vi "VGF Data.vi"(10 "Data":T1, 11 "Accion":enum16{"Read", "Set_data"}(ring)) -> (2 "Data 2":T1)   [LabVIEW 2019, in "Analisis.lvlib"]
doc: "FGV dedicated to storage momentarily the data in the analisis interface. This data is obtained in SAVE_DB_SQLite module to storage in the database"
uses:
  Analisis.lvlib
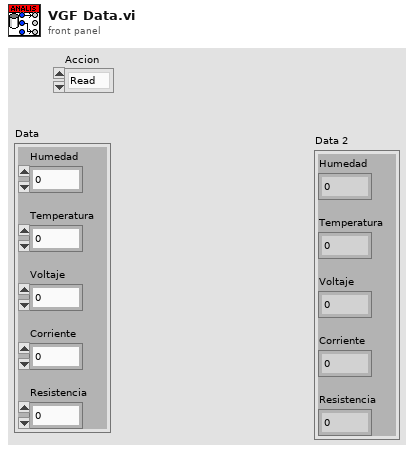
[diagram p1: front panel]
types:
  T1 = cluster{"Humedad":dbl, "Temperatura":dbl, "Voltaje":dbl, "Corriente":dbl, "Resistencia":i32}
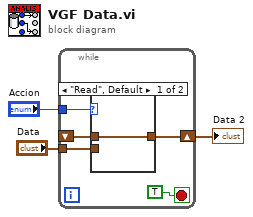
[diagram p0: block diagram]
diagram:
  n1 = while {
    tunnel: "Accion" -> [w8]
    tunnel: "Data" -> [w6]
    shift-right: [w5] -> w1
    shift-left: _ -> [w4]
    stop <- TRUE stop-if-true
    n2 = case shown="\"Read\", Default" w8 {
      tunnel: w6 -> [_ w10]
      tunnel: [w9 w10] -> w5
      tunnel: w4 -> [w9 _]
      frame "Read", Default {
      }
      frame "Set_data" {
      }
    }
  }
  "Data 2" <- w1
